vi "Parse Response.vi"(8 "error in (no error)":errorcluster, 10 "JSON String":string, 11 "Request":refnum<class "Request.lvclass">) -> (0 "error out":errorcluster, 1 "id":string, 2 "result":variant, 3 "Request out":refnum<class "Request.lvclass">)   [LabVIEW 2019, in "Request.lvclass"]
uses:
  Request.lvclass
  typedefs/JSON-RPC-Response Object--Cluster.ctl
  typedefs/Error Object--Cluster.ctl
  lv-venv/lv.lib/vi.lib/addons/_JKI.lib/Serialization/JSON/JKI JSON Serialization.lvlib
  JSON-RPC.lvclass
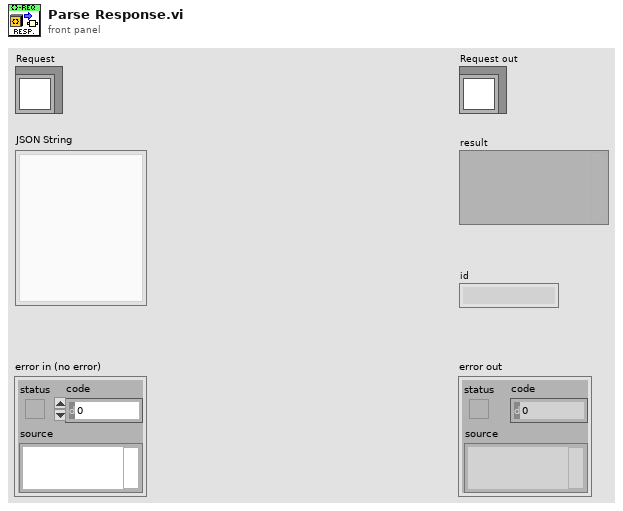
[diagram p1: front panel]
types:
  T1 = typedef "JSON-RPC.lvclass/Error Object--Cluster.ctl" = cluster{"code":i32, "message":string, "data":variant}
  T2 = typedef "JSON-RPC.lvclass/JSON-RPC-Response Object--Cluster.ctl" = cluster{"jsonrpc":string, "result":variant, "error":variant, "id":string}
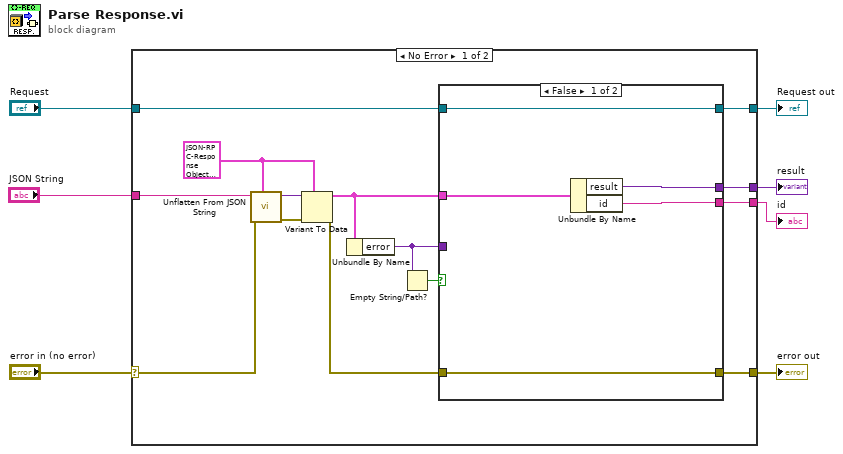
[diagram p0: block diagram]
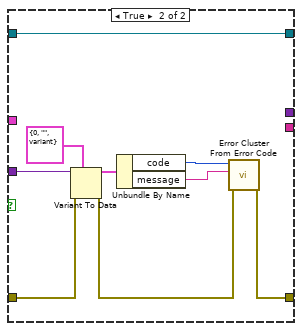
[diagram p2: hidden frame]
diagram:
  n1 = case shown="No Error" "error in (no error)" {
    selector: "error in (no error)" -> [w19 w37]
    tunnel: [w12 w37] -> w6
    tunnel: [w16 w36] -> w4
    tunnel: "Request" -> [w15 w36]
    tunnel: "JSON String" -> [w21 _]
    tunnel: [w17 _] -> w2
    tunnel: [w9 _] -> w1
    frame No Error {
      w8 = T2 {"jsonrpc"="", "result"=variant, "error"=variant, "id"=""} ("response")
      n2 = call "Unflatten From JSON String.vi"("Type and Defaults"=w8, "error in (no error)"=w19, "JSON String"=w21) -> ("error out"=w18:errorcluster, "Variant"=w20:variant)  [unwired: 7 in]
      n3 = Variant To Data(error in=w18, type=w8, Variant=w20) -> (data=w14:T2, error out=w13:errorcluster)
      n4 = Unbundle By Name(w14) -> ("error"=w10:variant)
      n5 = Empty String/Path?(string/path=w10) -> (empty?=w11:bool)
      n6 = case shown="False" w11 {
        tunnel: [w24 _] -> w17
        tunnel: [w26 w27] -> w16
        tunnel: w15 -> [w26 w27]
        tunnel: w14 -> [w25 _]
        tunnel: w10 -> [_ w35]
        tunnel: w13 -> [w23 w33]
        tunnel: [w23 w29] -> w12
        tunnel: [w22 _] -> w9
        frame False {
          n7 = Unbundle By Name(w25) -> ("result"=w24:variant, "id"=w22:string)
        }
        frame True {
          n8 = Variant To Data(error in=w33, type=T1 {"code"=0, "message"="", "data"=variant} ("Error"), Variant=w35) -> (data=w34:T1, error out=w30:errorcluster)
          n9 = Unbundle By Name(w34) -> ("code"=w32:i32, "message"=w31:string)
          n10 = call <vilib>:"Error Cluster From Error Code.vi"("error in (no error)"=w30, "error message (\"\")"=w31, "error code (0)"=w32) -> ("error out"=w29:errorcluster)  [unwired: 6 in]
        }
      }
    }
    frame Error {
    }
  }
  "error out" <- w6
  "Request out" <- w4
  "result" <- w2
  "id" <- w1
